vi "4145 set txt colour.vi"() -> ()   [LabVIEW 2014]
panel:
  out "length":i32
  in  "Boolean":bool
  in  "OK Button":bool
  out "Status":string
  in  "text end":u32
  in  "text start":u32
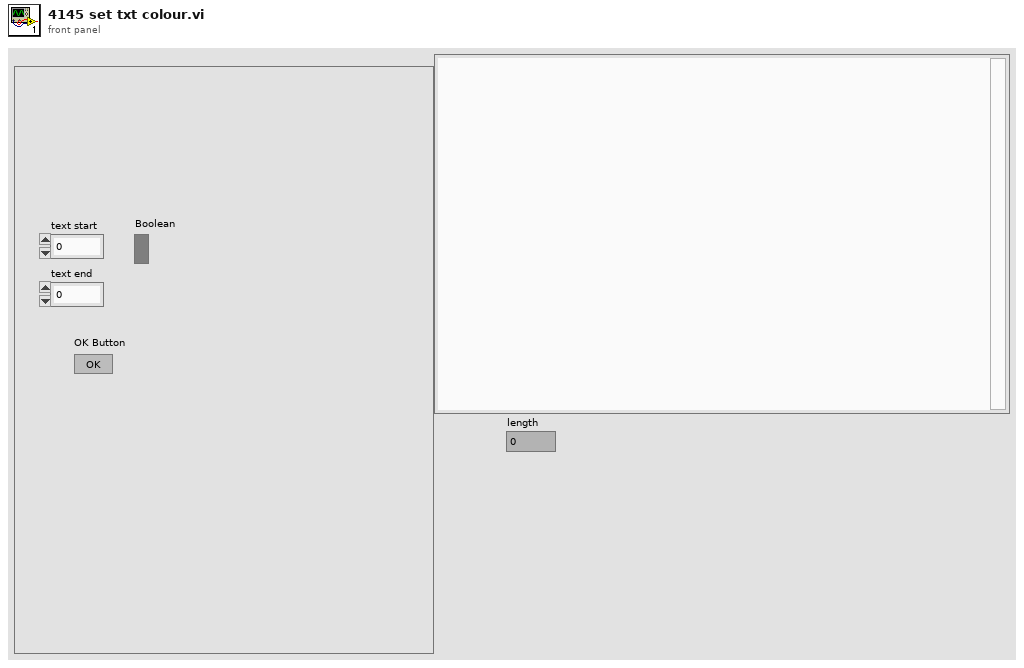
[diagram p1: front panel]
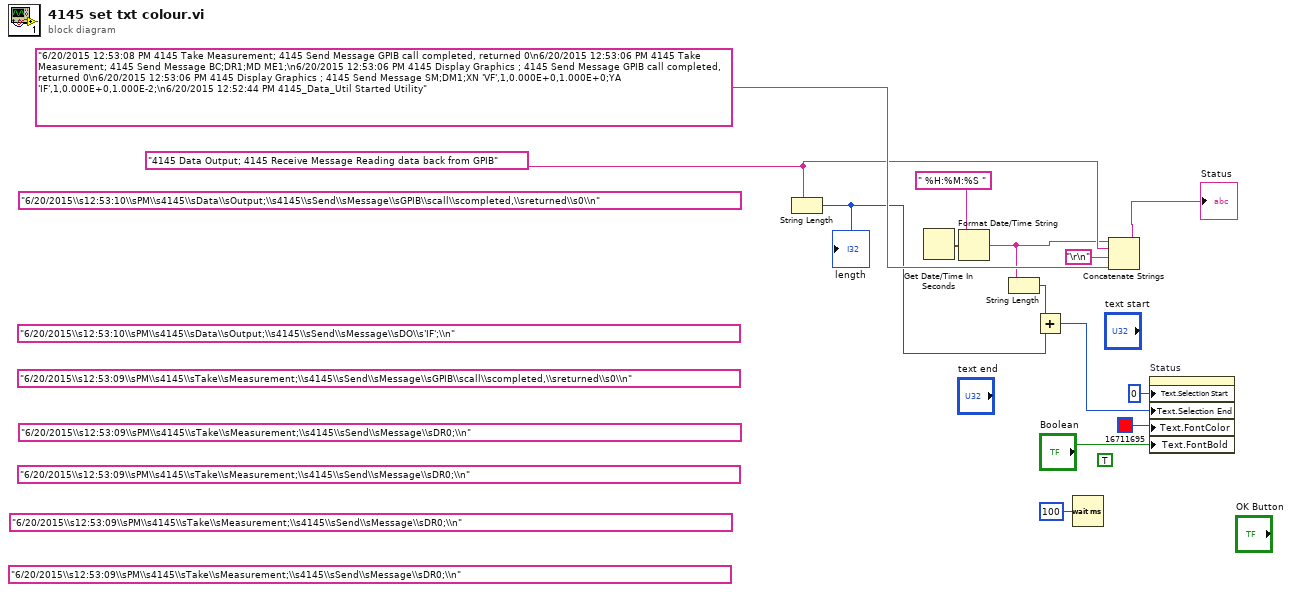
[diagram p0: block diagram]
diagram:
  (unwired) TRUE ("Text.Font:Bold")
  (unwired) "6/20/2015\\s12:53:09\\sPM\\s4145\\sTake\\sMeasurement;\\s4145\\sSend\\sMessage\\sDR0;\\n"
  (unwired) "6/20/2015\\s12:53:09\\sPM\\s4145\\sTake\\sMeasurement;\\s4145\\sSend\\sMessage\\sDR0;\\n"
  (unwired) "6/20/2015\\s12:53:09\\sPM\\s4145\\sTake\\sMeasurement;\\s4145\\sSend\\sMessage\\sDR0;\\n"
  (unwired) "6/20/2015\\s12:53:09\\sPM\\s4145\\sTake\\sMeasurement;\\s4145\\sSend\\sMessage\\sDR0;\\n"
  (unwired) "6/20/2015\\s12:53:09\\sPM\\s4145\\sTake\\sMeasurement;\\s4145\\sSend\\sMessage\\sGPIB\\scall\\scompleted,\\sreturned\\s0\\n"
  (unwired) "6/20/2015\\s12:53:10\\sPM\\s4145\\sData\\sOutput;\\s4145\\sSend\\sMessage\\sDO\\s'IF';\\n"
  (unwired) "6/20/2015\\s12:53:10\\sPM\\s4145\\sData\\sOutput;\\s4145\\sSend\\sMessage\\sGPIB\\scall\\scompleted,\\sreturned\\s0\\n"
  w7 = "4145 Data Output; 4145 Receive Message Reading data back from GPIB"
  n1 = String Length(string=w7) -> (length=w3:i32)
  "length" <- w3
  n2 = Get Date/Time In Seconds() -> (seconds since 1Jan1904=w9:timestamp)
  n3 = Format Date/Time String(time format string (%c)=" %H:%M:%S ", seconds (now)=w9) -> (date/time string=w5:string)  [unwired: 1 in]
  n4 = String Length(string=w5) -> (length=w4:i32)
  n5 = Add(x=w4, y=w3) -> (x+y=w2:i32)
  n6 = Wait (ms)(milliseconds to wait=u32 100) -> ()  [unwired: 1 out]
  n7 = Concatenate Strings(w5, w7, "\r\n", "6/20/2015 12:53:08 PM 4145 Take Measurement; 4145 Send Message GPIB call completed, returned 0\n6/20/2015 12:53:06 PM 4145 Take Measurement; 4145 Send Message BC;DR1;MD ME1;\n6/20/2015 12:53:06 PM 4145 Display Graphics ; 4145 Send Message GPIB call completed, returned 0\n6/20/2015 12:53:06 PM 4145 Display Graphics ; 4145 Send Message SM;DM1;XN 'VF',1,0.000E+0,1.000E+0;YA 'IF',1,0.000E+0,1.000E-2;\n6/20/2015 12:52:44 PM 4145_Data_Util Started Utility") -> (→"Status":string)
  n8 = property on="Status" class="Str"("Text.Selection Start"=u32 0 ("Text.Selection:Start"), "Text.Selection End"=w2, "Text.FontColor"=u32 16711695, "Text.FontBold"="Boolean") -> ()  [unwired: 2 in, 2 out]
